vi "FreeMemory_CopyDataToCPU.vi"(1 "Array Dst In Host":u8[](array[numeric]), 4 "Error IN Toolkit":i32, 5 "Error In LabVIEW":errorcluster) -> (15 "Array Dst OUT Host":u8[](array[numeric]), 18 "Error OUT Toolkit":i32, 19 "Error Out LabVIEW":errorcluster)   [LabVIEW 2018]
doc: "It copies in an 1D Array U8 stored in CPU the results of an 1D U8 array stored in GPU and frees GPU memory of the Array. It receives an 1D U8 array.\n\nFor correct operation it should receive an error that comes from a VI of some processing algorithm."
uses:
  dll/LibreriaAutis_3.dll
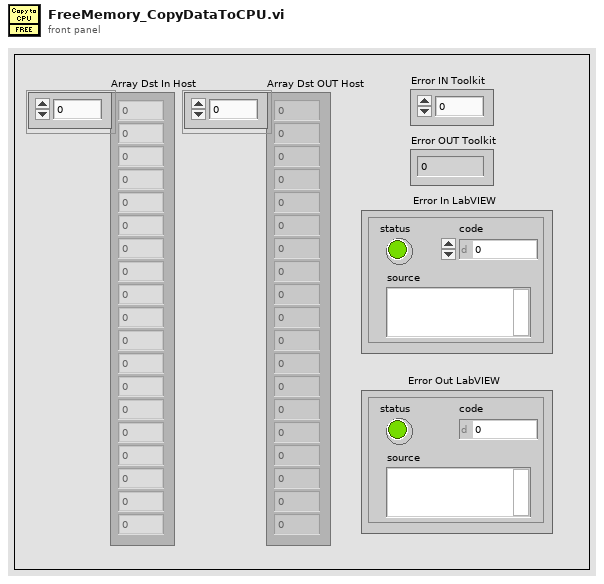
[diagram p1: front panel]
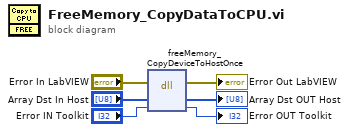
[diagram p0: block diagram]
diagram:
  n1 = dll-call lib="C:/Users/AUTIS/Desktop/LibreriaAUTIS/LabVIEW/dll/LibreriaAutis_3.dll" fn="freeMemory_CopyDeviceToHostOnce"(error in="Error In LabVIEW", "dst"="Array Dst In Host", "error"="Error IN Toolkit") -> (error out=→"Error Out LabVIEW":errorcluster, "dst"=→"Array Dst OUT Host":u8[], "error"=→"Error OUT Toolkit":i32)  [unwired: 3 in, 1 out]
